vi "oa_SCL Scale XY Data.vi"(1 "y scale factors":cluster{"a":dbl, "b":dbl, "log?":bool} {"b" format="%.2f"; "a" format="%.2f"}, 2 "x scale factors":cluster{"a":dbl, "b":dbl, "log?":bool} {"b" format="%.2f"; "a" format="%.2f"}, 3 "xy data":cluster{"x":dbl, "y":dbl}[](array[cluster]) {"y" format="%.2f"; "x" format="%.2f"}) -> (0 "scaled xy data":cluster{"x":i16, "y":i16}[](array[cluster]))   [LabVIEW 2017]
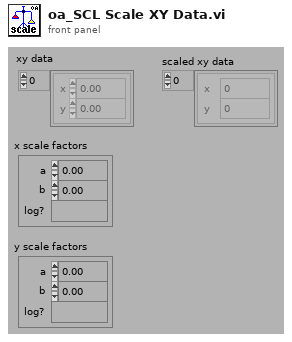
[diagram p1: front panel]
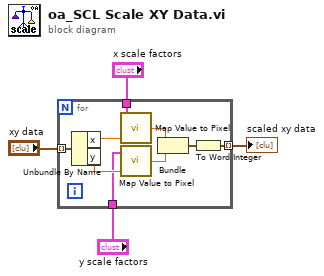
[diagram p0: block diagram]
diagram:
  n1 = for {
    tunnel: "xy data" -> [w13] mode=indexing
    tunnel: "x scale factors" -> [w11]
    tunnel: "y scale factors" -> [w8]
    tunnel: [w5] -> w1 mode=indexing
    n2 = Unbundle By Name(w13) -> ("x"=w12:dbl, "y"=w9:dbl)
    n3 = call <vilib>:"Map Value to Pixel.vi"("x"=w12, "scale factors"=w11) -> ("pixel"=w10:dbl)  [unwired: 1 in]
    n4 = call <vilib>:"Map Value to Pixel.vi"("x"=w9, "scale factors"=w8) -> ("pixel"=w7:dbl)  [unwired: 1 in]
    n5 = Bundle("pixel"=w10, "pixel"=w7) -> (w6:cluster{"pixel":dbl, "pixel":dbl})  [unwired: 1 in]
    n6 = To Word Integer(number=w6) -> (16bit integer=w5:cluster{"pixel":i16, "pixel":i16})
  }
  "scaled xy data" <- w1
